vi "create_data_folders.vi"(6 "Application Directory":string, 9 "Experiment Title":string, 10 "Username":string, 11 "Folderpath on C:":path) -> (3 "Folderpath on C: out":path)   [LabVIEW 2018]
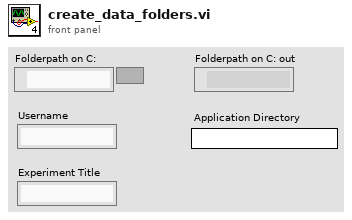
[diagram p1: front panel]
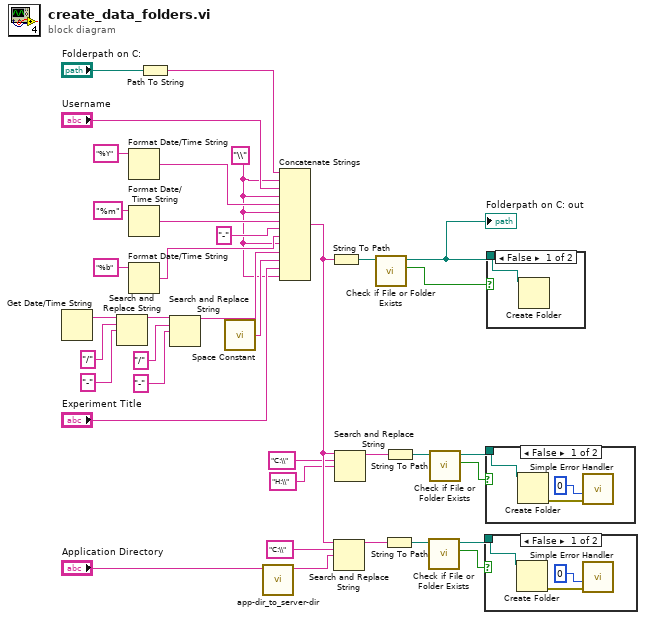
[diagram p0: block diagram]
diagram:
  w5 = "\\"
  n1 = Get Date/Time String() -> (date string=w23:string)  [unwired: 3 in, 1 out]
  n2 = Search and Replace String(input string=w23, search string="/", replace string="-") -> (result string=w33:string)  [unwired: 5 in, 3 out]
  n3 = Format Date/Time String(time format string (%c)="%Y") -> (date/time string=w13:string)  [unwired: 2 in]
  n4 = Format Date/Time String(time format string (%c)="%m") -> (date/time string=w14:string)  [unwired: 2 in]
  n5 = Format Date/Time String(time format string (%c)="%b") -> (date/time string=w15:string)  [unwired: 2 in]
  n6 = Path To String(path="Folderpath on C:") -> (string=w3:string)
  n7 = Search and Replace String(input string=w33, search string="/", replace string="-") -> (result string=w34:string)  [unwired: 5 in, 3 out]
  n8 = call <vilib>:"Space Constant.vi"() -> ("String"=w35:string)
  n9 = call "app-dir_to_server-dir.vi"("Application Directory"="Application Directory") -> ("Group Server Directory"=w2:string)  [unwired: 10 in]
  n10 = Concatenate Strings(w3, w5, "Username", w5, w13, w5, w14, "-", w15, w5, w34, w35, "Experiment Title", w5) -> (w37:string)
  n11 = String To Path(string=w37) -> (path=w8:path)
  n12 = Search and Replace String(input string=w37, search string="C:\\", replace string=w2) -> (result string=w30:string)  [unwired: 5 in, 3 out]
  n13 = Search and Replace String(input string=w37, search string="C:\\", replace string="H:\\") -> (result string=w26:string)  [unwired: 5 in, 3 out]
  n14 = call <vilib>:"Check if File or Folder Exists.vi"("path"=w8) -> ("file or folder exists?"=w7:bool, "dup path"=w6:path)  [unwired: 8 in, 1 out]
  "Folderpath on C: out" <- w6
  n15 = String To Path(string=w30) -> (path=w22:path)
  n16 = String To Path(string=w26) -> (path=w19:path)
  n17 = call <vilib>:"Check if File or Folder Exists.vi"("path"=w22) -> ("file or folder exists?"=w21:bool, "dup path"=w20:path)  [unwired: 8 in, 1 out]
  n18 = call <vilib>:"Check if File or Folder Exists.vi"("path"=w19) -> ("file or folder exists?"=w18:bool, "dup path"=w17:path)  [unwired: 8 in, 1 out]
  n19 = case shown="False" w21 {
    tunnel: w20 -> [w40 _]
    frame False {
      n20 = Create Folder(path (use dialog)=w40) -> (error out=w39:errorcluster)  [unwired: 2 in, 2 out]
      n21 = call <vilib>:"Simple Error Handler.vi"("type of dialog (OK msg:1)"=0, "error in (no error)"=w39) -> ()  [unwired: 3 in, 5 out]
    }
    frame True {
    }
  }
  n22 = case shown="False" w18 {
    tunnel: w17 -> [w43 _]
    frame False {
      n23 = Create Folder(path (use dialog)=w43) -> (error out=w42:errorcluster)  [unwired: 2 in, 2 out]
      n24 = call <vilib>:"Simple Error Handler.vi"("type of dialog (OK msg:1)"=0, "error in (no error)"=w42) -> ()  [unwired: 3 in, 5 out]
    }
    frame True {
    }
  }
  n25 = case shown="False" w7 {
    tunnel: w6 -> [w44 _]
    frame False {
      n26 = Create Folder(path (use dialog)=w44) -> ()  [unwired: 2 in, 3 out]
    }
    frame True {
    }
  }
